vi "Configure.vi"(8 "error in (no error)":errorcluster, 11 "Laser_Oxxius in":refnum<class "Laser_Oxxius.lvclass">) -> (0 "error out":errorcluster, 3 "Laser_Oxxius out":refnum<class "Laser_Oxxius.lvclass">)   [LabVIEW 2020, in "Laser_Oxxius.lvlib" / "Laser_Oxxius.lvclass"]
uses:
  Laser_Oxxius.lvclass
  E:/Development/DevHardSoftware/MMicroscopyAF/Model/HAL Layer/Component/Device/Device/Device.lvclass
  Laser_Oxxius.lvclass/Laser_Oxxius.ctl
  HAL Layer/Component/Laser/Laser/Laser.lvclass
  HAL Layer/Component/Device/Device/Device.lvclass
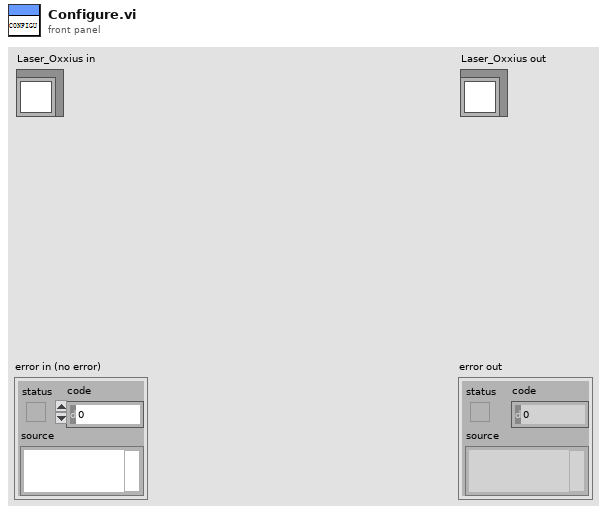
[diagram p1: front panel]
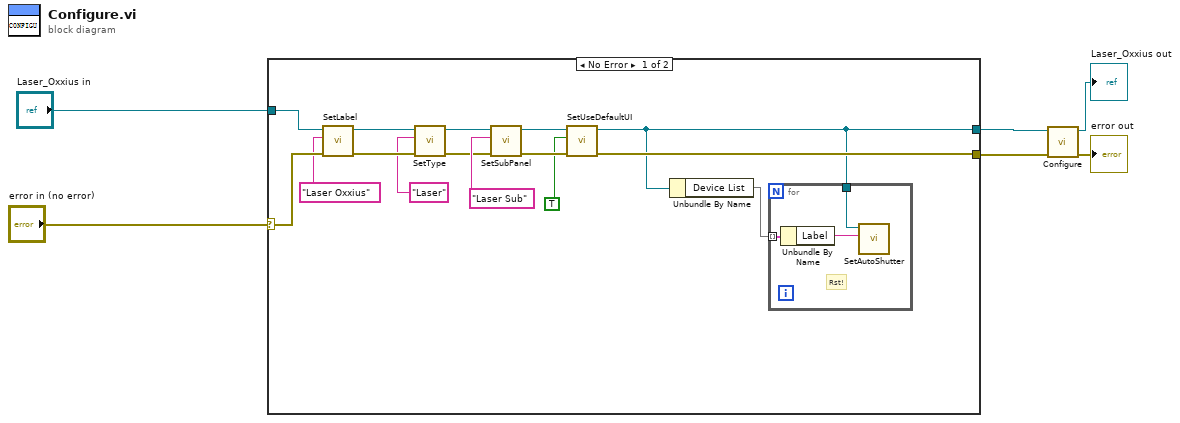
[diagram p0: block diagram]
diagram:
  n1 = case shown="No Error" "error in (no error)" {
    selector: "error in (no error)" -> [w20 w26]
    tunnel: [w9 w26] -> w1
    tunnel: [w7 w25] -> w2
    tunnel: "Laser_Oxxius in" -> [w21 w25]
    frame No Error {
      n2 = call-dynamic "SetLabel.vi"("error in (no error)"=w20, "Label"="Laser Oxxius", "Device in"=w21) -> ("error out"=w17:errorcluster, "Device out"=w18:refnum<class "Laser_Oxxius.lvclass">)  [unwired: 7 in]
      n3 = call-dynamic "SetType.vi"("error in (no error)"=w17, "Type"="Laser", "Device in"=w18) -> ("error out"=w10:errorcluster, "Device out"=w11:refnum<class "Laser_Oxxius.lvclass">)  [unwired: 7 in]
      n4 = call-dynamic "SetSubPanel.vi"("error in (no error)"=w10, "Sub Panel"="Laser Sub", "Device in"=w11) -> ("error out"=w15:errorcluster, "Device out"=w13:refnum<class "Laser_Oxxius.lvclass">)  [unwired: 7 in]
      n5 = call "SetUseDefaultUI.vi"("error in (no error)"=w15, "Use Default UI?"=TRUE, "Device in"=w13) -> ("error out"=w9:errorcluster, "Device out"=w7:refnum<class "Laser_Oxxius.lvclass">)  [unwired: 7 in]
      n6 = Unbundle By Name(w7) -> ("Device List"=w8:map{string, refnum<k24>})
      n7 = for {
        tunnel: w8 -> [w24] mode=indexing
        tunnel: w7 -> [w22]
        # "Rst!"
        n8 = Unbundle By Name(w24) -> ("Label"=w23:string)
        n9 = call-dynamic "SetAutoShutter.vi"("Label"=w23, "Laser_Oxxius in"=w22) -> ()  [unwired: 8 in, 2 out]
      }
    }
    frame Error {
    }
  }
  n10 = call-parent "Configure.vi"("error in (no error)"=w1, "Device in"=w2) -> ("error out"=→"error out":errorcluster, "Device out"=→"Laser_Oxxius out":refnum<class "Laser_Oxxius.lvclass">)  [unwired: 8 in]
